vi "Apply Gain & Offset (1D).vi"(8 "Number of Bits":i16=14, 9 "Offset":dbl, 10 "Range (V)":dbl=2.07, 11 "Raw Data":i16[](array[numeric])) -> (3 "Scaled Data":dbl[](array[numeric]) format="%.2f")   [LabVIEW 2012]
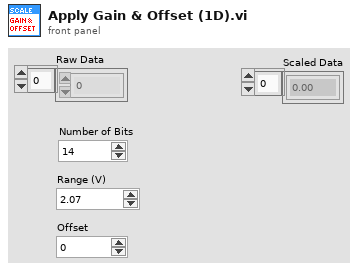
[diagram p1: front panel]
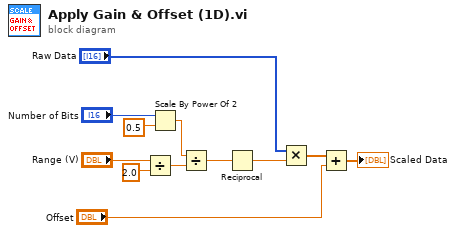
[diagram p0: block diagram]
diagram:
  n1 = Divide(x="Range (V)", y=2.0) -> (x/y=w3:dbl)
  n2 = Scale By Power Of 2(n="Number of Bits", x=0.5) -> (x*2^n=w6:dbl)
  n3 = Divide(x=w6, y=w3) -> (x/y=w5:dbl)
  n4 = Reciprocal(x=w5) -> (1/x=w1:dbl)
  n5 = Multiply(x="Raw Data", y=w1) -> (x*y=w11:dbl[])
  n6 = Add(x=w11, y="Offset") -> (x+y=→"Scaled Data":dbl[])
